vi "Unflatten I2C Linux Header.vi"(8 "error in (no error)":errorcluster, 10 "Bytes in":u8[](array[numeric]), 11 "pcap Parse and Build in":refnum<class "pcap Parse and Build.lvclass">) -> (0 "error out":errorcluster, 1 "I2C Lunix Header Out":T1, 2 "Bytes out":u8[](array[numeric]), 3 "pcap Parse and Build out":refnum<class "pcap Parse and Build.lvclass">)   [LabVIEW 2021, in "pcap Parse and Build.lvclass"]
uses:
  pcap Parse and Build.lvclass
  Typedef/I2C Linux Header.ctl
  pcap Parse and Build.lvclass/pcap Parse and Build.ctl
  Typedef/Errors.ctl
  241affe9-119b-4122-8cbe-bc40c9af6f32.vi
  241affe9-119b-4122-8cbe-bc40c9af6f32.vi/c28b0ead-42ad-4072-80a2-aca7f2bd7ce3.vi
  <vilib>/CIF Foundation/CIF Utilities/Errors/Append Error Location.vi
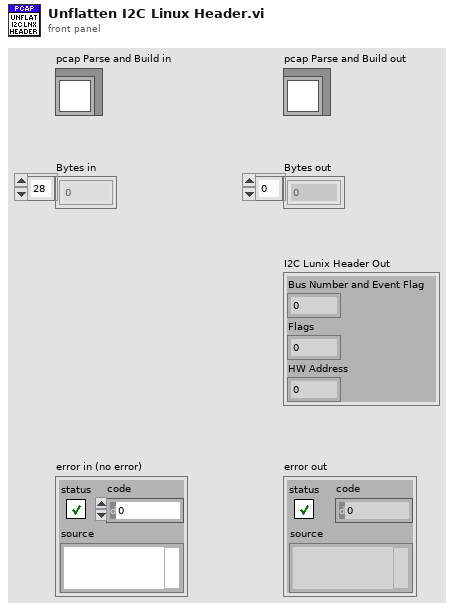
[diagram p1: front panel]
types:
  T1 = typedef "pcap Parse and Build.lvclass/I2C Linux Header.ctl" = cluster{"Bus Number and Event Flag":u8, "Flags":u32, "HW Address":u8}
  T2 = typedef "pcap Parse and Build.lvclass/Errors.ctl" = enum16{"Invalid Global Header", "Out of Data"}
  T3 = typedef "DataTypes_CIF_U.lvlib/Endian.ctl" = enum16{"Little Endian", "Big Endian"}
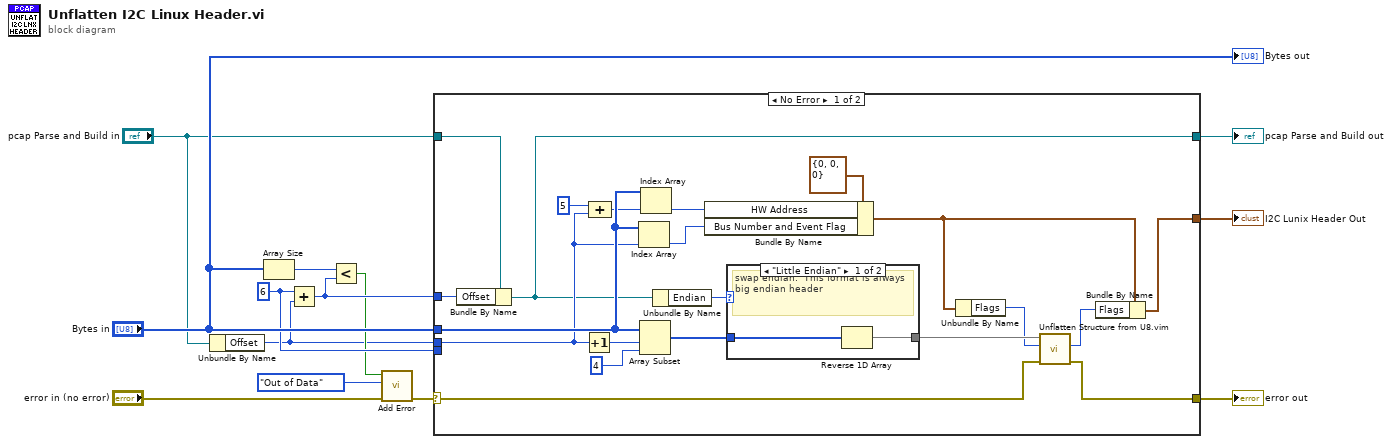
[diagram p0: block diagram]
diagram:
  w11 = 6 ("length")
  n1 = Unbundle By Name("pcap Parse and Build in") -> ("Offset"=w4:i32)
  n2 = Array Size(array="Bytes in") -> (size(s)=w6:i32)
  n3 = Add(x=w11, y=w4) -> (x+y=w12:i32)
  n4 = Less?(x=w6, y=w12) -> (x < y?=w10:bool)
  n5 = call "Add Error.vi"("error in (no error)"="error in (no error)", "Error"=Errors."Out of Data", "Insert Error"=w10) -> ("error out"=w7:errorcluster)  [unwired: 8 in]
  n6 = case shown="No Error" w7 {
    selector: w7 -> [w33 w39]
    tunnel: [w34 w39] -> w5
    tunnel: "Bytes in" -> [w24 _]
    tunnel: w12 -> [w31 _]
    tunnel: w11 -> [_ _]
    tunnel: w4 -> [w23 _]
    tunnel: "pcap Parse and Build in" -> [w32 w38]
    tunnel: [w18 w38] -> w2
    tunnel: [w14 _] -> w1
    frame No Error {
      n7 = Bundle By Name(cluster=w32, "Offset"=w31) -> (w18:refnum<class "pcap Parse and Build.lvclass">)
      n8 = Increment(x=w23) -> (x+1=w26:i32)
      n9 = Compound Arithmetic op=ADD(5 ("value"), w23) -> (w22:i32)
      n10 = Index Array(array=w24, index=w23) -> (element=w19:u8)
      n11 = Array Subset(array=w24, index=w26, length=4) -> (w30:u8[])
      n12 = Index Array(array=w24, index=w22) -> (element=w20:u8)
      n13 = Unbundle By Name(w18) -> ("Endian"=w28:T3)
      n14 = Bundle By Name(cluster=T1 {"Bus Number and Event Flag"=0, "Flags"=0, "HW Address"=0} ("I2C Linux Header out"), "HW Address"=w20, "Bus Number and Event Flag"=w19) -> (w15:T1)
      n15 = case shown="\"Little Endian\"" w28 {
        tunnel: w30 -> [w36 w37]
        tunnel: [w35 w37] -> w29
        frame "Little Endian" {
          # "swap endian.  This format is always big endian header"
          n16 = Reverse 1D Array(array=w36) -> (reversed array=w35:u8[])
        }
        frame "Big Endian" {
        }
      }
      n17 = Unbundle By Name(w15) -> ("Flags"=w17:u32)
      n18 = call "Unflatten Structure from U8.vim"("error in"=w33, "Type"=w17, "Flattend Data in"=w29) -> ("error out"=w34:errorcluster, "Unflattend Data"=w16:u32)  [unwired: 6 in, 1 out]
      n19 = Bundle By Name(cluster=w15, "Flags"=w16) -> (w14:T1)
    }
    frame Error {
    }
  }
  "pcap Parse and Build out" <- w2
  "error out" <- w5
  "I2C Lunix Header Out" <- w1
  "Bytes out" <- "Bytes in"
